vi "Second VI.vi"(9 "Numero echant":i32=8, 11 "Array":dbl[](array[numeric])) -> (1 "Array 2":dbl[](array[numeric]))   [LabVIEW 2013]
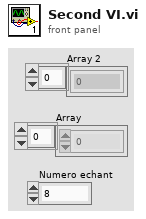
[diagram p1: front panel]
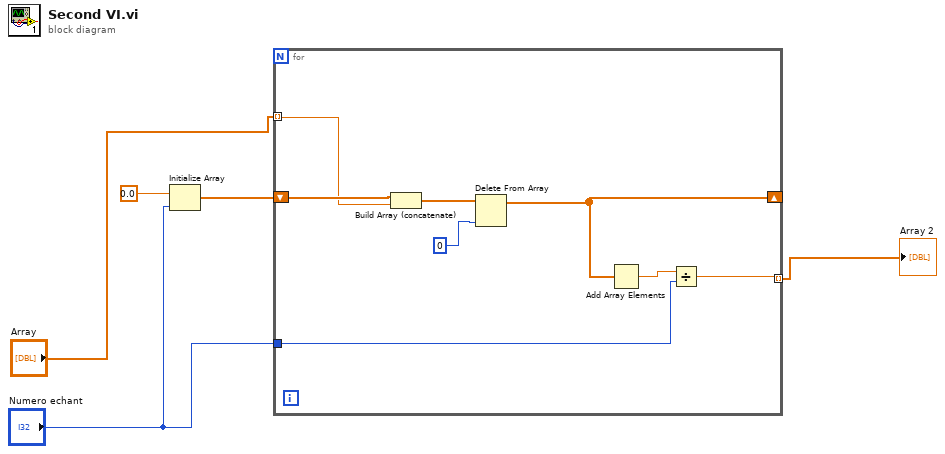
[diagram p0: block diagram]
diagram:
  n1 = Initialize Array(0.0, "Numero echant") -> (w4:dbl[])
  n2 = for {
    shift-right: [w7] -> _
    shift-left: w4 -> [w13]
    tunnel: "Array" -> [w12] mode=indexing
    tunnel: [w10] -> w1 mode=indexing
    tunnel: "Numero echant" -> [w9]
    n3 = Build Array (concatenate)(w13, w12) -> (w6:dbl[])
    n4 = Delete From Array(array=w6, index=0) -> (array with subset deleted=w7:dbl[])  [unwired: 1 in, 1 out]
    n5 = Add Array Elements(numeric array=w7) -> (sum=w11:dbl)
    n6 = Divide(x=w11, y=w9) -> (x/y=w10:dbl)
  }
  "Array 2" <- w1
